vi "Arduino generic wrapper.vi"(2 "Tx msg cluster":T1={"dest"=1, "A/D/C/I"="A", "R/W"="R", "chan"=1, "val (float)"=0.0}, 3 "Port name":string) -> (0 "Scan comment":string, 1 "Output":dbl)   [LabVIEW 2013]
uses:
  ctls_and_globals/Arduino tx msg cluster.ctl
  ctls_and_globals/Arduino Config & resource typedef.ctl
  ctls_and_globals/Arduino Global.vi
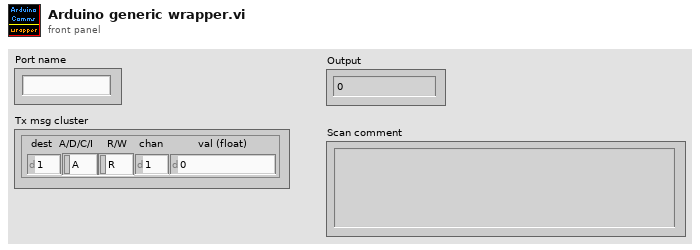
[diagram p1: front panel]
types:
  T1 = typedef "Arduino tx msg cluster.ctl" = cluster{"dest":u8, "A/D/C/I":string, "R/W":string, "chan":u8, "val (float)":sgl}
  T2 = typedef "Arduino Config & resource typedef.ctl" = cluster{"VISA resource name":refnum<visa-resource-name>, "baud rate (bps)":u32, "timeout (ms)":u32, "data bits":u16, "parity":enum16{"None", "Odd", "Even", "Mark", "Space"}, "stop bits (10: 1 bit)":u16, "flow control":u16, "termination char (hex)":u8, "Enable Termination Char":bool, "byte count":u32, "Resource locked?":bool}
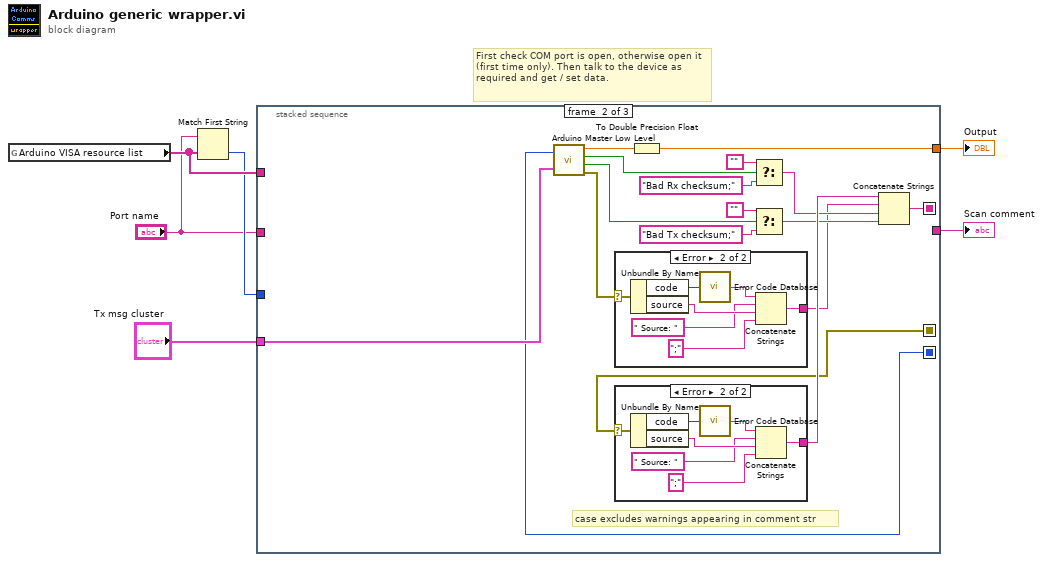
[diagram p0: block diagram]
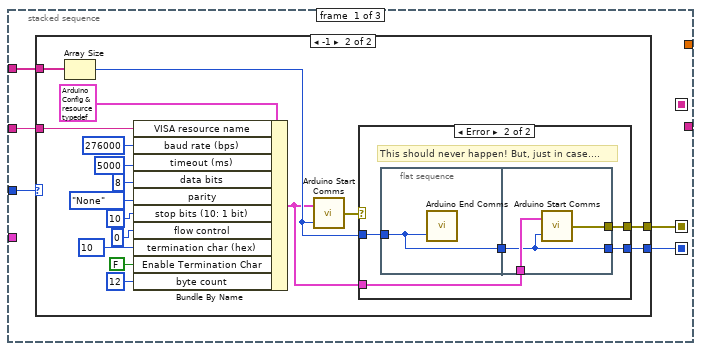
[diagram p2: hidden frame]
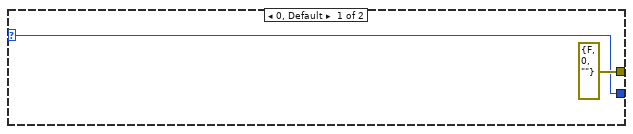
[diagram p3: hidden frame]
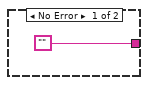
[diagram p5: hidden frame]
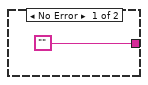
[diagram p6: hidden frame]
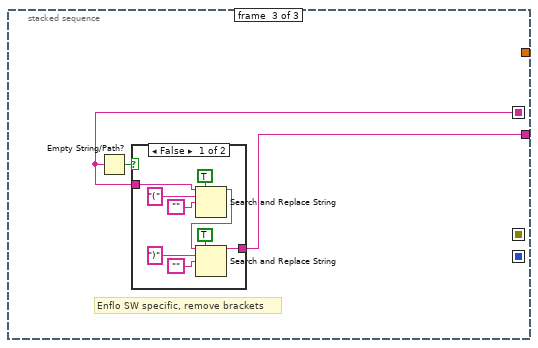
[diagram p7: hidden frame]
diagram:
  # "First check COM port is open, otherwise open it (first time only). Then talk to the device as required and get / set data."
  n1 = global read "Arduino Global.vi" "Arduino VISA resource list"() -> (w6:string[])
  n2 = Match First String(2:w6, 3:"Port name") -> (0:w5:i32)  [unwired: 1 out]
  n3 = stacked-sequence {
    seq-local: [w8 _ _] -> [_ w47 _]
    seq-local: [w7 _ _] -> [_ w45 _]
    seq-local: [_ w42 _] -> [_ _ w76]
    tunnel: w5 -> [w11 _ _]
    tunnel: w6 -> [w10 _ _]
    tunnel: "Port name" -> [w9 _ _]
    tunnel: [_ w57 _] -> w4
    tunnel: "Tx msg cluster" -> [_ w46 _]
    tunnel: [_ _ w75] -> w1
    frame #0 {
      n4 = case shown="-1" w11 {
        selector: w11 -> [w12 _]
        tunnel: w10 -> [_ w30]
        tunnel: w9 -> [_ w28]
        tunnel: [errorcluster {"status"=FALSE, "code"=0, "source"=""} ("Error") w15] -> w8
        tunnel: [w12 w14] -> w7
        frame 0, Default {
        }
        frame -1 {
          n5 = Array Size(array=w30) -> (size(s)=w17:i32)
          n6 = Bundle By Name(cluster=T2 {"VISA resource name"="COM12", "baud rate (bps)"=276000, "timeout (ms)"=5000, "data bits"=8, "parity"=enum."None", "stop bits (10: 1 bit)"=10, "flow control"=0, "termination char (hex)"=10, "Enable Termination Char"=FALSE, "byte count"=12, "Resource locked?"=FALSE} ("Arduino VISA config & resource"), "VISA resource name"=w28, "baud rate (bps)"=u32 276000, "timeout (ms)"=u32 5000, "data bits"=u16 8, "parity"=enum16{"None", "Odd", "Even", "Mark", "Space"}."None", "stop bits (10: 1 bit)"=u16 10, "flow control"=u16 0, "termination char (hex)"=u8 10, "Enable Termination Char"=FALSE, "byte count"=u32 12) -> (w16:T2)
          n7 = call "Arduino Start Comms.vi"("Resource index"=w17, "Arduino VISA config & resource"=w16) -> ("Error"=w18:errorcluster)
          n8 = case shown="Error" w18 {
            selector: w18 -> [w32 _]
            tunnel: w17 -> [w31 w37]
            tunnel: w16 -> [_ w36]
            tunnel: [w32 w34] -> w15
            tunnel: [w31 w33] -> w14
            frame No Error {
            }
            frame Error {
              # "This should never happen! But, just in case...."
              n9 = flat-sequence {
                tunnel: w37 -> [w38]
                tunnel: [w38] -> w35
                tunnel: w36 -> [w41]
                tunnel: w35 -> [w39]
                tunnel: [w40] -> w34
                tunnel: [w39] -> w33
                frame #0 {
                  n10 = call "Arduino End Comms.vi"("Resource index"=w38) -> ()  [unwired: 2 out]
                }
                frame #1 {
                  n11 = call "Arduino Start Comms.vi"("Resource index"=w39, "Arduino VISA config & resource"=w41) -> ("Error"=w40:errorcluster)
                }
              }
            }
          }
        }
      }
    }
    frame #1 {
      # "case excludes warnings appearing in comment str"
      n12 = call "Arduino Master Low Level.vi"("Arduino VISA resource index"=w45, "Tx msg cluster"=w46) -> ("Value returned"=w58:sgl, "Rx checksum ok?"=w56:bool, "Tx checksum ok?"=w55:bool, "Error"=w44:errorcluster)
      n13 = case shown="Error" w44 {
        selector: w44 -> [_ w65]
        tunnel: ["" w66] -> w43
        frame No Error {
        }
        frame Error {
          n14 = Unbundle By Name(w65) -> ("code"=w64:i32, "source"=w61:string)
          n15 = call <vilib>:"Error Code Database.vi"("Error Code"=w64) -> ("Error Text"=w63:string)
          n16 = Concatenate Strings(w63, " Source: " ("string"), w61, ";") -> (w66:string)
        }
      }
      n17 = case shown="Error" w47 {
        selector: w47 -> [_ w73]
        tunnel: ["" w74] -> w50
        frame No Error {
        }
        frame Error {
          n18 = Unbundle By Name(w73) -> ("code"=w72:i32, "source"=w69:string)
          n19 = call <vilib>:"Error Code Database.vi"("Error Code"=w72) -> ("Error Text"=w71:string)
          n20 = Concatenate Strings(w71, " Source: " ("string"), w69, ";") -> (w74:string)
        }
      }
      n21 = To Double Precision Float(number=w58) -> (double precision float=w57:dbl)
      n22 = Select(t="", s=w56, f="Bad Rx checksum;") -> (s? t:f=w49:string)
      n23 = Select(t="", s=w55, f="Bad Tx checksum;") -> (s? t:f=w48:string)
      n24 = Concatenate Strings(w50, w43, w49, w48) -> (w42:string)
    }
    frame #2 {
      # "Enflo SW specific, remove brackets"
      n25 = Empty String/Path?(string/path=w76) -> (empty?=w77:bool)
      n26 = case shown="False" w77 {
        tunnel: w76 -> [w79 w87]
        tunnel: [w78 w87] -> w75
        frame False {
          n27 = Search and Replace String(replace all?=TRUE ("replace all? (F)"), input string=w79, search string="(", replace string="") -> (result string=w80:string)  [unwired: 4 in, 3 out]
          n28 = Search and Replace String(replace all?=TRUE ("replace all? (F)"), input string=w80, search string=")", replace string="") -> (result string=w78:string)  [unwired: 4 in, 3 out]
        }
        frame True {
        }
      }
    }
  }
  "Output" <- w4
  "Scan comment" <- w1
